vi "Restart opCRD.vi"(8 "error in":errorcluster, 11 "tCRD in":refnum<class "Open Path CRD.lvclass">) -> (0 "error out":errorcluster, 3 "tCRD out":refnum<class "Open Path CRD.lvclass">)   [LabVIEW 2015, in "Open Path CRD.lvclass"]
uses:
  Open Path CRD.lvclass
  <vilib>/nisyscfg/nisyscfg.lvlib
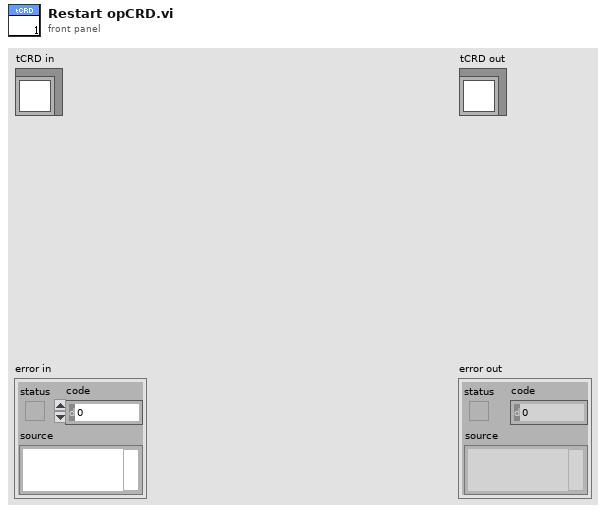
[diagram p1: front panel]
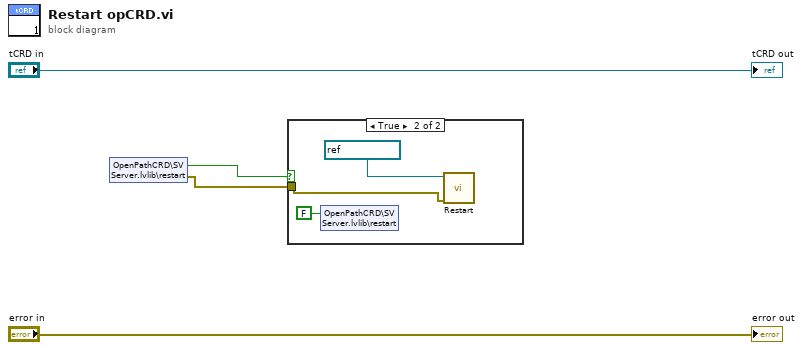
[diagram p0: block diagram]
diagram:
  n1 = shared-variable "OpenPathCRD\\SV Server.lvlib\\restart"() -> (w2:bool, error out=w1:errorcluster)  [unwired: 1 in]
  n2 = case shown="True" w2 {
    tunnel: w1 -> [_ w6]
    frame False {
    }
    frame True {
      n3 = shared-variable "OpenPathCRD\\SV Server.lvlib\\restart"(FALSE ("restart")) -> ()  [unwired: 1 in, 1 out]
      n4 = call <vilib>:"Restart.vi"("error in (no error)"=w6, "Session in"=refnum<k21> "localhost") -> ()  [unwired: 7 in, 3 out]
    }
  }
  "error out" <- "error in"
  "tCRD out" <- "tCRD in"
